vi "Station Config.vi"(8 "error in":errorcluster) -> (0 "error out":errorcluster)   [LabVIEW 2025, in "Full User Interface.lvlib"]
uses:
  Full User Interface.lvlib
  Station Config.ctl
  Station Info.ctl
  Localization/Section.ctl
  Localization/Localization.lvlib
panel:
  in  "Cancel":bool
  in  "OK":bool
  in  "Tree":string(tree)
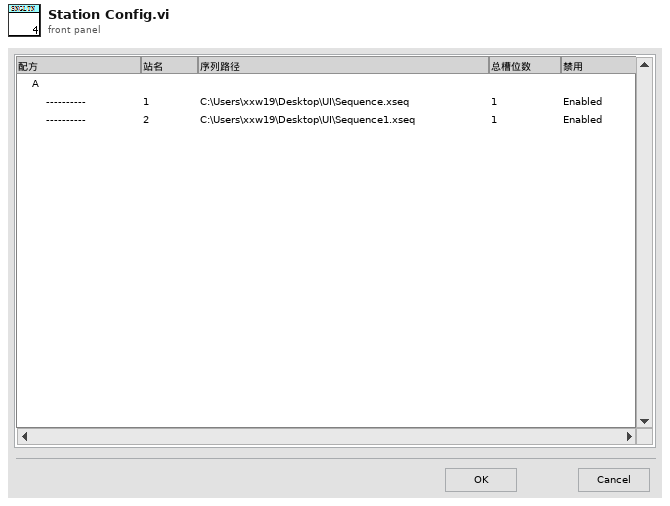
[diagram p1: front panel]
types:
  T1 = enum32{"Invalid", "Standard", "Closed", "Hidden", "Minimized", "Maximized"}
  T2 = enum32{"invalid app kind", "Development System", "Run Time System", "Student Edition", "Embedded LabVIEW", "Evaluation", "Custom"}
  T3 = typedef "Localization.lvlib/Section.ctl" = enum16{"Menu", "Title", "Workstation Config", "TestInterface"}
  T4 = cluster{"Navigate Tree:Get Parent":string, "Tag":string, "Col":i32}
  T5 = typedef "LVPoint32TypeDef.ctl" = cluster{"Horizontal":i32, "Vertical":i32}
  T6 = typedef "Full User Interface.lvlib/Station Config.ctl" = map{string, map{i32, T7}}
  T7 = typedef "Full User Interface.lvlib/Station Info.ctl" = cluster{"SeqFilename":path, "NumberOfSocket":i32, "Disable":bool}
  T8 = cluster{"Core":cluster{"Current VI Reference":refnum<vi>, "Close Panel on Exit?":bool}, "Tree":refnum<vi>, "Station Config":T6, "variant":variant, "clipboard":map{i32, T7}}
  T9 = cluster{"Current VI Reference":refnum<vi>, "Close Panel on Exit?":bool}
  T10 = cluster{"Left Cell String":string, "Child Text":string[], "Child Tag":string, "Item Indent":i32, "Child Only?":bool, "Glyph Index":i32}[]
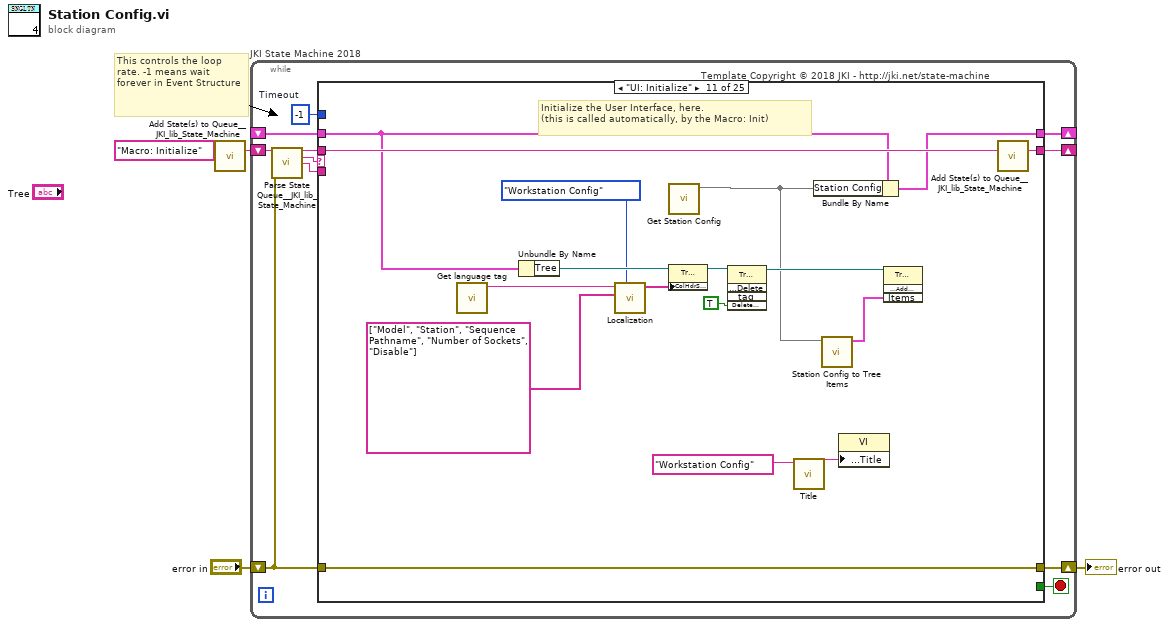
[diagram p0: block diagram]
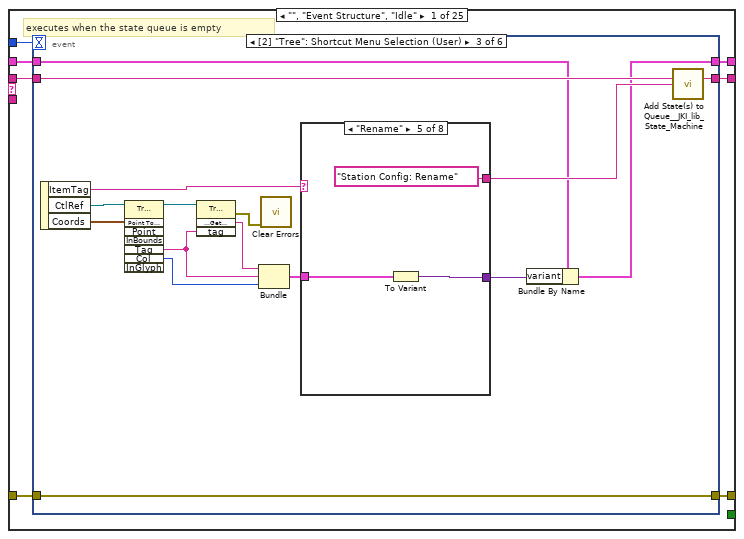
[diagram p2: hidden frame]
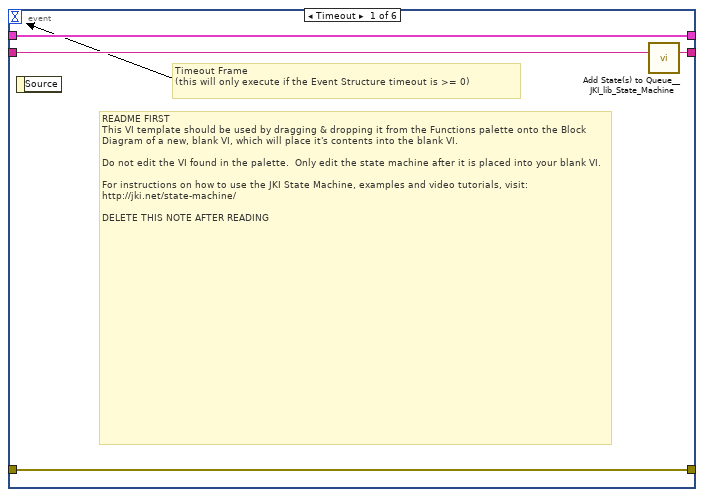
[diagram p3: hidden frame]
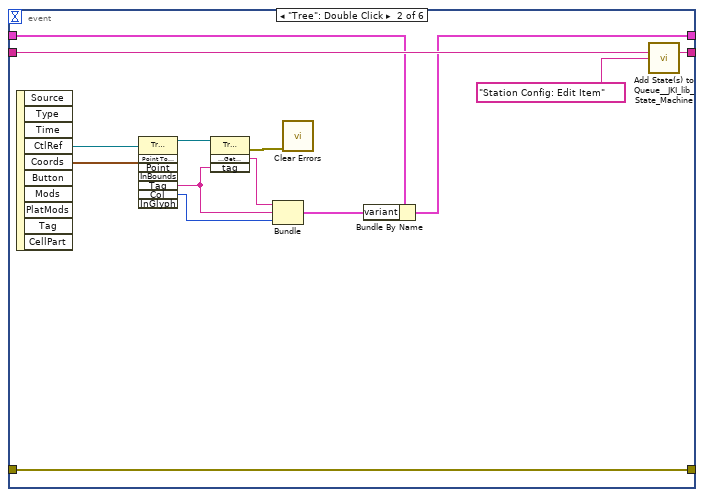
[diagram p4: hidden frame]
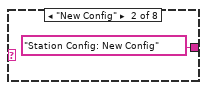
[diagram p6: hidden frame]
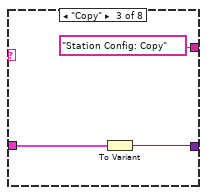
[diagram p7: hidden frame]
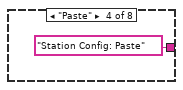
[diagram p8: hidden frame]
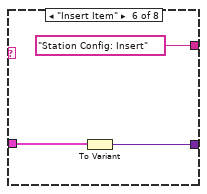
[diagram p9: hidden frame]
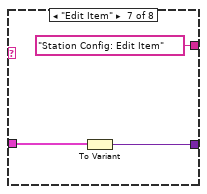
[diagram p10: hidden frame]
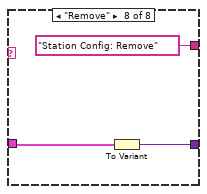
[diagram p11: hidden frame]
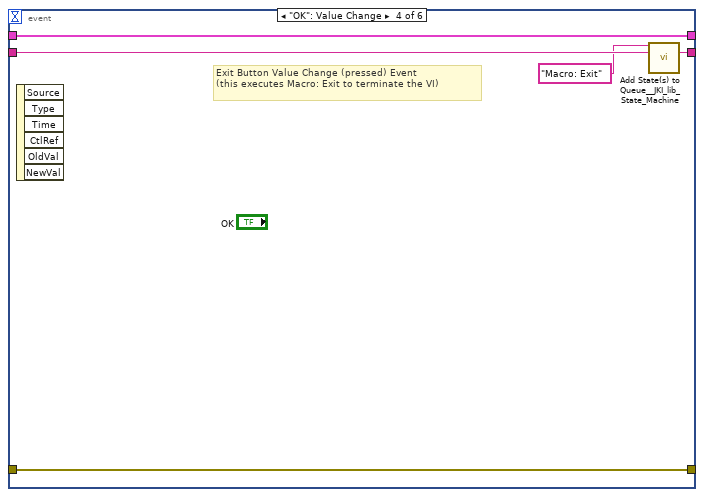
[diagram p12: hidden frame]
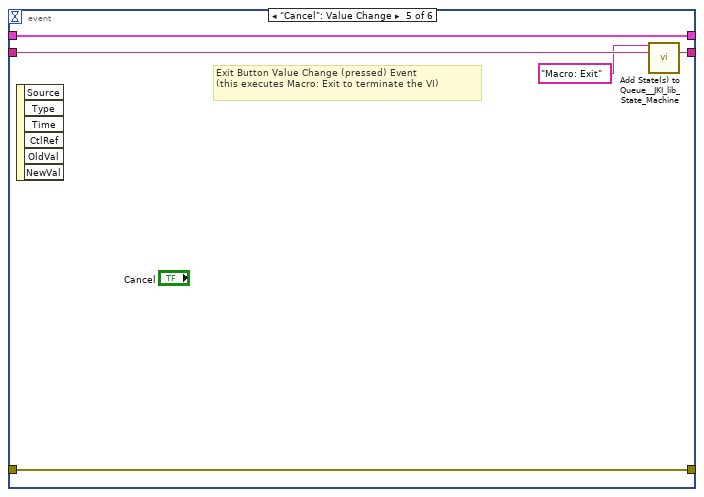
[diagram p13: hidden frame]
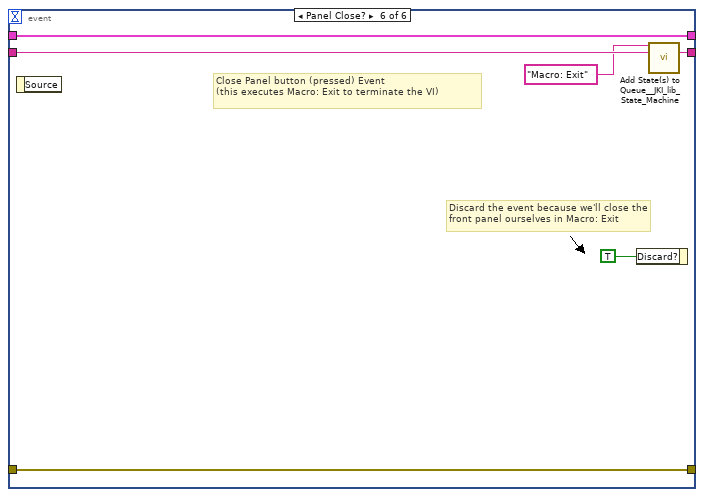
[diagram p14: hidden frame]
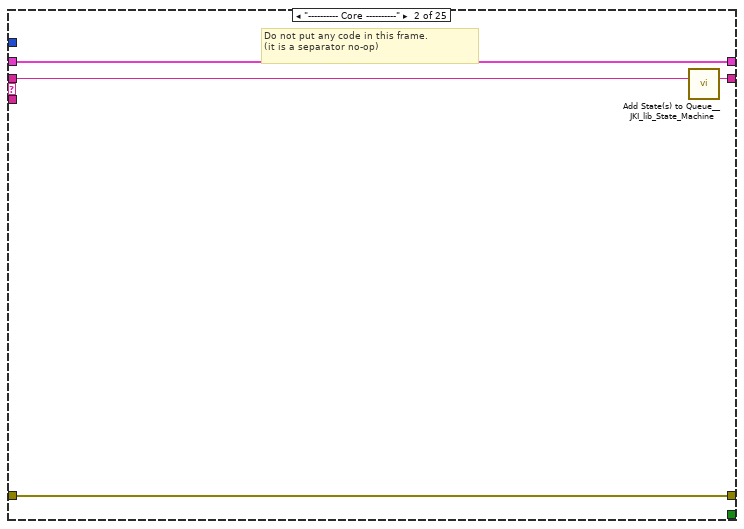
[diagram p15: hidden frame]
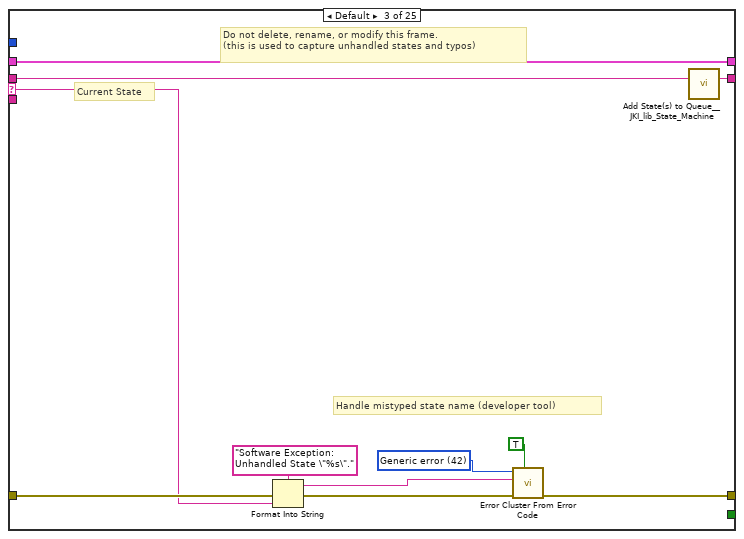
[diagram p16: hidden frame]
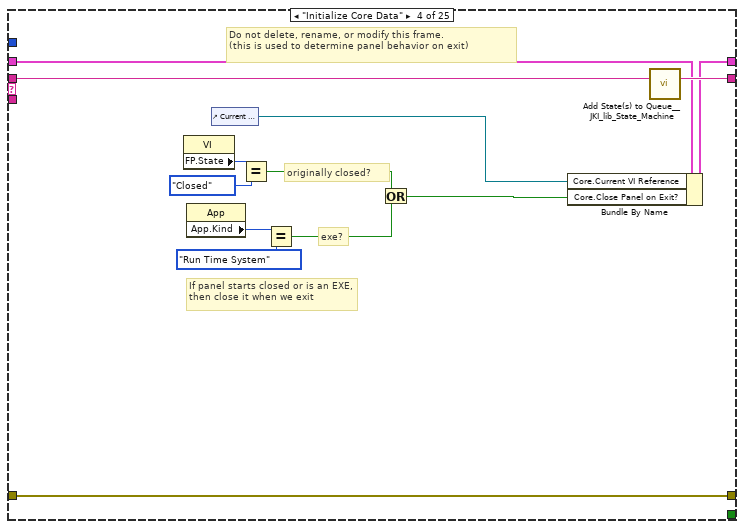
[diagram p17: hidden frame]
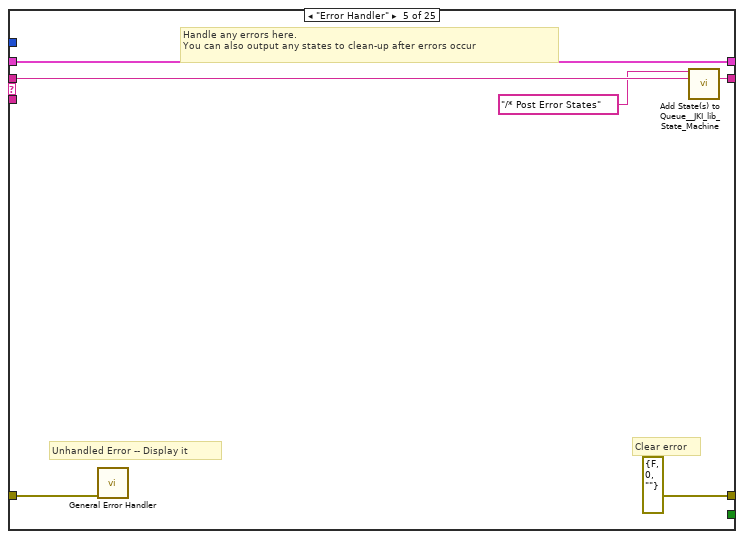
[diagram p18: hidden frame]
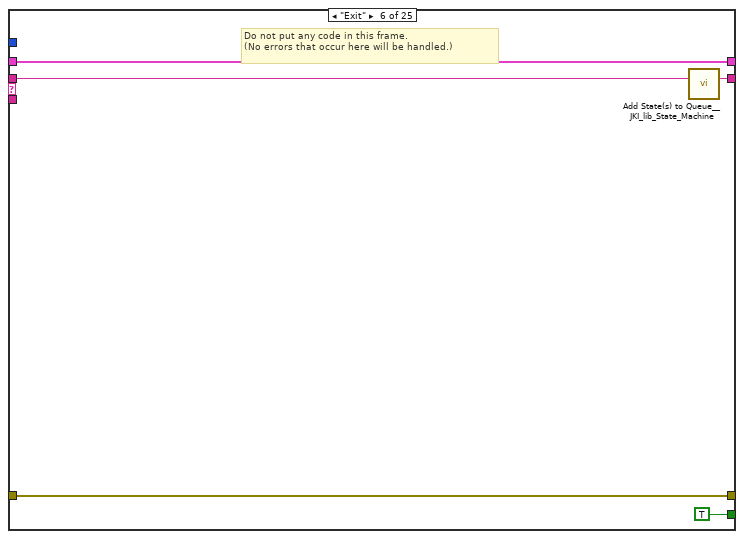
[diagram p19: hidden frame]
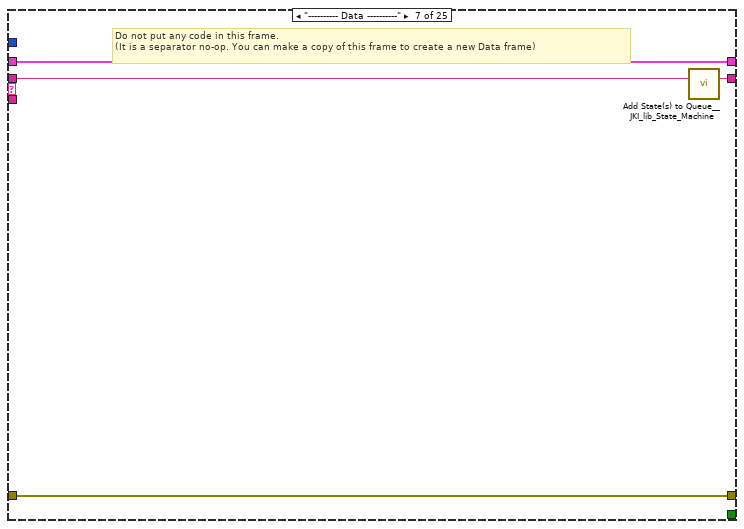
[diagram p20: hidden frame]
diagram:
  # "This controls the loop rate. -1 means wait forever in Event Structure"
  n1 = call <vilib>:"Add State(s) to Queue__JKI_lib_State_Machine.vi"("State(s) in (\"\")"="Macro: Initialize") -> ("States Out"=w4:string)  [unwired: 14 in]
  n2 = while "JKI State Machine 2018" {
    shift-right: [w8] -> _
    shift-left: _ -> [w7]
    shift-right: [w11] -> w1
    shift-left: "error in" -> [w5]
    shift-right: [w10] -> _
    shift-left: w4 -> [w12]
    stop <- w9 stop-if-true
    w6 = -1  # Timeout
    # "Template Copyright © 2018 JKI - http://jki.net/state-machine"
    n3 = call <vilib>:"Parse State Queue__JKI_lib_State_Machine.vi"("State Queue"=w12, "Error In (no error)"=w5) -> ("Remaining States"=w14:string, "Current State"=w15:string, "Arguments"=w13:string)  [unwired: 11 in]
    n4 = case shown="\"UI: Initialize\"" w15 {
      selector: w15 -> [_ _ w94 _ _ _ _ _ _ _ _ _ _ _ _ _ _ _ _ _ _ _ _ _ _]
      tunnel: w14 -> [w22 w93 w98 w117 w123 w128 w132 w141 w147 w151 w168 w174 w185 w254 w259 w269 w273 w280 w288 w303 w319 w335 w345 w354 w377]
      tunnel: w13 -> [_ _ _ _ _ _ _ _ _ _ _ w169 w179 _ _ _ _ _ _ _ _ _ _ _ _]
      tunnel: w7 -> [w20 w90 w96 w110 w120 w126 w129 _ w142 w148 w162 w172 w181 w251 w256 w266 w270 w277 w284 w292 w308 w328 w338 w349 w369]
      tunnel: [w19 w91 w100 w114 errorcluster {"status"=FALSE, "code"=0, "source"=""} ("error out") w125 w130 w138 w143 w149 w166 w170 w182 w252 w257 w267 w271 w275 w286 w301 w317 w333 w343 w352 w375] -> w11
      tunnel: w5 -> [w18 w91 w99 w114 w119 w125 w130 w138 w144 w149 w166 w171 w183 w252 w257 w267 w271 w278 w286 w301 w317 w333 w343 w352 w375]
      tunnel: [w21 w92 w97 w116 w122 w127 w131 w140 w146 w150 w167 w173 w184 w253 w258 w268 w272 w279 w287 w302 w318 w334 w344 w353 w376] -> w10
      tunnel: [_ _ _ _ _ TRUE _ _ _ _ _ _ _ _ _ _ _ _ _ _ _ _ _ _ _] -> w9
      tunnel: [w17 w90 w96 w115 w120 w126 w129 w139 w142 w148 w160 w172 w181 w251 w256 w266 w270 w277 w282 w290 w306 w326 w336 w348 w367] -> w8
      tunnel: w6 -> [w16 _ _ _ _ _ _ _ _ _ _ _ _ _ _ _ _ _ _ _ _ _ _ _ _]
      frame "", "Event Structure", "Idle" {
        # "executes when the state queue is empty"
        n5 = event shown="[2] \"Tree\": Shortcut Menu Selection (User)" {
          selector: _ -> [_ _ _ _ _ _]
          dyn-events: _ -> [_ _ _ _ _ _]
          timeout: w16 -> [_ _ _ _ _ _]
          tunnel: w22 -> [w26 w40 w56 w78 w83 w89]
          tunnel: [w25 w39 w55 w77 w82 w88] -> w21
          tunnel: w20 -> [w23 w29 w47 w75 w80 w86]
          tunnel: [w24 w38 w54 w76 w81 w87] -> w19
          tunnel: w18 -> [w24 w38 w54 w76 w81 w87]
          tunnel: [w23 w28 w46 w75 w80 w86] -> w17
          event Timeout {
            # "README FIRST\nThis VI template should be used by dragging & dropping it from the Functions palette onto the Block Diagram of a new, blank VI, which will place it's contents into the blank VI.\n\nDo not edit the VI found in the palette.  Only edit the state machine after it is placed into your blank VI.\n\nFor instructions on how to use the JKI State Machine, examples and video tutorials, visit:\nhttp://jki.net/state-machine/\n\nDELETE THIS NOTE AFTER READING"
            # "Timeout Frame\n(this will only execute if the Event Structure timeout is >= 0)"
            n6 = event-data() -> ()  [unwired: 1 in, 1 out]
            n7 = call <vilib>:"Add State(s) to Queue__JKI_lib_State_Machine.vi"("State(s) in (\"\")"=w26) -> ("States Out"=w25:string)  [unwired: 14 in]
          }
          event "Tree": Double Click {
            n8 = event-data() -> ("CtlRef"=w32:refnum<vi>, "Coords"=w31:T5)  [unwired: 1 in, 8 out]
            n9 = invoke class="Tree (strict)" method="Point To Row Column"(reference=w32, "Point"=w31) -> (reference out=w36:refnum<vi>, "Tag"=w35:string, "Col"=w37:i32)  [unwired: 6 in, 5 out]
            n10 = invoke class="Tree (strict)" method="Navigate Tree.Get Parent"(reference=w36, "tag"=w35) -> (error out=w33:errorcluster, "Navigate Tree:Get Parent"=w34:string)  [unwired: 2 in, 2 out]
            n11 = Bundle("Navigate Tree:Get Parent"=w34, "Tag"=w35, "Col"=w37) -> (w30:T4)  [unwired: 1 in]
            n12 = call <vilib>:"Clear Errors.vi"("error in (no error)"=w33) -> ()  [unwired: 5 in, 2 out]
            n13 = Bundle By Name(cluster=w29, "variant"=w30) -> (w28:T8)
            n14 = call <vilib>:"Add State(s) to Queue__JKI_lib_State_Machine.vi"("State(s) in (\"\")"=w40, "State(s) at Back (\"\")"="Station Config: Edit Item" ("State(s) at Back (\"\")")) -> ("States Out"=w39:string)  [unwired: 13 in]
          }
          event "Tree": Shortcut Menu Selection (User) {
            n15 = event-data() -> ("ItemTag"=w53:string, "CtlRef"=w52:refnum<vi>, "Coords"=w51:T5)  [unwired: 1 in]
            n16 = invoke class="Tree (strict)" method="Point To Row Column"(reference=w52, "Point"=w51) -> (reference out=w44:refnum<vi>, "Tag"=w43:string, "Col"=w49:i32)  [unwired: 6 in, 5 out]
            n17 = invoke class="Tree (strict)" method="Navigate Tree.Get Parent"(reference=w44, "tag"=w43) -> (error out=w41:errorcluster, "Navigate Tree:Get Parent"=w42:string)  [unwired: 2 in, 2 out]
            n18 = Bundle("Navigate Tree:Get Parent"=w42, "Tag"=w43, "Col"=w49) -> (w48:T4)  [unwired: 1 in]
            n19 = call <vilib>:"Clear Errors.vi"("error in (no error)"=w41) -> ()  [unwired: 5 in, 2 out]
            n20 = case shown="\"Rename\"" w53 {
              tunnel: [_ "Station Config: New Config" "Station Config: Copy" "Station Config: Paste" "Station Config: Rename" "Station Config: Insert" "Station Config: Edit Item" "Station Config: Remove"] -> w50
              tunnel: w48 -> [_ _ w59 _ w63 w66 w69 w72]
              tunnel: [_ _ w58 _ w62 w65 w68 w71] -> w45
              frame Default {
              }
              frame "New Config" {
              }
              frame "Copy" {
                n21 = To Variant(anything=w59) -> (Variant=w58:variant)
              }
              frame "Paste" {
              }
              frame "Rename" {
                n22 = To Variant(anything=w63) -> (Variant=w62:variant)
              }
              frame "Insert Item" {
                n23 = To Variant(anything=w66) -> (Variant=w65:variant)
              }
              frame "Edit Item" {
                n24 = To Variant(anything=w69) -> (Variant=w68:variant)
              }
              frame "Remove" {
                n25 = To Variant(anything=w72) -> (Variant=w71:variant)
              }
            }
            n26 = Bundle By Name(cluster=w47, "variant"=w45) -> (w46:T8)
            n27 = call <vilib>:"Add State(s) to Queue__JKI_lib_State_Machine.vi"("State(s) in (\"\")"=w56, "State(s) at Back (\"\")"=w50) -> ("States Out"=w55:string)  [unwired: 13 in]
          }
          event "OK": Value Change {
            # "Exit Button Value Change (pressed) Event\n(this executes Macro: Exit to terminate the VI)"
            n28 = event-data() -> ()  [unwired: 1 in, 6 out]
            n29 = call <vilib>:"Add State(s) to Queue__JKI_lib_State_Machine.vi"("State(s) in Front (\"\")"="Macro: Exit", "State(s) in (\"\")"=w78) -> ("States Out"=w77:string)  [unwired: 13 in]
          }
          event "Cancel": Value Change {
            # "Exit Button Value Change (pressed) Event\n(this executes Macro: Exit to terminate the VI)"
            n30 = event-data() -> ()  [unwired: 1 in, 6 out]
            n31 = call <vilib>:"Add State(s) to Queue__JKI_lib_State_Machine.vi"("State(s) in Front (\"\")"="Macro: Exit", "State(s) in (\"\")"=w83) -> ("States Out"=w82:string)  [unwired: 13 in]
          }
          event Panel Close? {
            # "Discard the event because we'll close the front panel ourselves in Macro: Exit"
            # "Close Panel button (pressed) Event\n(this executes Macro: Exit to terminate the VI)"
            n32 = event-data() -> ()  [unwired: 1 in, 1 out]
            n33 = event-data("Discard?"=TRUE) -> ()  [unwired: 1 in, 1 out]
            n34 = call <vilib>:"Add State(s) to Queue__JKI_lib_State_Machine.vi"("State(s) in Front (\"\")"="Macro: Exit", "State(s) in (\"\")"=w89) -> ("States Out"=w88:string)  [unwired: 13 in]
          }
        }
      }
      frame "---------- Core ----------" {
        # "Do not put any code in this frame.\n(it is a separator no-op)"
        n35 = call <vilib>:"Add State(s) to Queue__JKI_lib_State_Machine.vi"("State(s) in (\"\")"=w93) -> ("States Out"=w92:string)  [unwired: 14 in]
      }
      frame Default {
        w103 = 42 items=["No error", "Argument error", "Memory is full", "Out of zone", "End of file", "File already open", "Generic file I/O error", "File not found", "File permission error", "Disk is full", "Duplicate path", "Too many files open", "System feature not enabled", "Resource file not found", "Cannot add resource", "Resource not found", "Image not found", "Image memory error", "Pen does not exist", "Config type invalid", "Config token not found", "Config parse error", "Config memory error", "Bad external code format", "Bad external code offset", "External code not present", "Null window", "Destroy window error", "Null menu", "Print aborted", "Bad print record", "Print driver error", "Windows error during printing", "Memory error during printing", "Print dialog error", "Generic print error", "Invalid device refnum", "Device not found", "Device parameter error", "Device unit error", "Cannot open device", "Device call aborted", "Generic error", "Cancelled by user", "Object ID too low", "Object ID too high", "Object not in heap", "Unknown heap", "Unknown object (invalid DefProc)", "Unknown object (DefProc not in table)", "Message out of range", "Invalid (null) method", "Unknown message", "Manager call not supported", "Bad address", "Network operation in progress", "Network operation timed out", "Connection is busy", "Network attribute not supported", "Network error", "Address in use", "System out of memory", "Connection aborted", "Connection refused", "Not connected", "Already connected", "Connection closed", "Initialization error (interapplication manager)", "Bad occurrence", "Wait on unbound occurrence handler", "Occurrence queue overflow", "Datalog type conflict", "Unused", "Unrecognized type (interapplication manager)", "Memory corrupt", "Failed to make temporary DLL", "Old CIN version", "Drag socket not found", "Failed to load drop-object", "Failed to register OLE object", "Failed to release OLE object", "Format specifier type mismatch", "Unknown format specifier", "Too few format specifiers", "Too many format specifiers", "Scan failed", "Newer CIN version", "Error converting to variant", "Runtime menu error", "Password tampered", "Variant attribute not found", "Incompatible variant data type", "Event data is not available", "Event Store is not present", "Occurrence is not found", "Event Queue is not created", "Event info is not available", "Refnum passed is NULL", "Error retrieving Class GUID", "Error retrieving CoClass GUID", "Error retrieving TypeLib GUID.", "Bad built application magic bytes.", "Specific driver is different from the specific driver associated with the Logical Name.", "There is no session opened to the class driver.", "Max Error", "MAX - Error with config objects", "MAX - Error loading configuration", "MAX - Group not supported"]
        # "Current State"
        # "Do not delete, rename, or modify this frame.\n(this is used to capture unhandled states and typos)"
        # "Handle mistyped state name (developer tool)"
        n36 = Format Into String(format string="Software Exception: Unhandled State \"%s\"." ("message"), error in=w99, w94) -> (resulting string=w102:string, error out=w101:errorcluster)  [unwired: 1 in]
        n37 = call <vilib>:"Error Cluster From Error Code.vi"("show call chain? (False)"=TRUE, "error in (no error)"=w101, "error message (\"\")"=w102, "error code (0)"=w103) -> ("error out"=w100:errorcluster)  [unwired: 5 in]
        n38 = call <vilib>:"Add State(s) to Queue__JKI_lib_State_Machine.vi"("State(s) in (\"\")"=w98) -> ("States Out"=w97:string)  [unwired: 14 in]
      }
      frame "Initialize Core Data" {
        # "Do not delete, rename, or modify this frame.\n(this is used to determine panel behavior on exit)"
        # "originally closed?"
        # "exe?"
        # "If panel starts closed or is an EXE, then close it when we exit"
        n39 = property class="VI"() -> ("FP.State"=w107:T1)  [unwired: 2 in, 2 out]
        n40 = property class="App"() -> ("App.Kind"=w113:T2)  [unwired: 2 in, 2 out]
        n41 = control-ref of="Current VI Reference"() -> (w108:refnum<vi>)
        n42 = Equal?(x=w107, y=T1."Closed" ("Front Panel Window:State")) -> (x = y?=w105:bool)
        n43 = Equal?(x=w113, y=T2."Run Time System" ("Application:Kind")) -> (x = y?=w111:bool)
        n44 = Or(x=w105, y=w111) -> (x .or. y?=w109:bool)
        n45 = Bundle By Name(cluster=w110, "Core.Current VI Reference"=w108, "Core.Close Panel on Exit?"=w109) -> (w115:T8)
        n46 = call <vilib>:"Add State(s) to Queue__JKI_lib_State_Machine.vi"("State(s) in (\"\")"=w117) -> ("States Out"=w116:string)  [unwired: 14 in]
      }
      frame "Error Handler" {
        # "Unhandled Error -- Display it"
        # "Handle any errors here.\nYou can also output any states to clean-up after errors occur"
        # "Clear error"
        n47 = call <vilib>:"General Error Handler.vi"("error in (no error)"=w119) -> ()  [unwired: 10 in, 5 out]
        n48 = call <vilib>:"Add State(s) to Queue__JKI_lib_State_Machine.vi"("State(s) in Front (\"\")"="/* Post Error States", "State(s) in (\"\")"=w123) -> ("States Out"=w122:string)  [unwired: 13 in]
      }
      frame "Exit" {
        # "Do not put any code in this frame.\n(No errors that occur here will be handled.)"
        n49 = call <vilib>:"Add State(s) to Queue__JKI_lib_State_Machine.vi"("State(s) in (\"\")"=w128) -> ("States Out"=w127:string)  [unwired: 14 in]
      }
      frame "---------- Data ----------" {
        # "Do not put any code in this frame.\n(It is a separator no-op. You can make a copy of this frame to create a new Data frame)"
        n50 = call <vilib>:"Add State(s) to Queue__JKI_lib_State_Machine.vi"("State(s) in (\"\")"=w132) -> ("States Out"=w131:string)  [unwired: 14 in]
      }
      frame "Data: Initialize" {
        w133 = map{i32, T7} {}  # clipboard
        w134 = variant  # variant
        w135 = T6 {}  # Station Config
        w137 = T9 {"Current VI Reference"=refnum, "Close Panel on Exit?"=FALSE}  # Core
        # "Data names and types of shift register data are defined by this bundle."
        # "Initialize the shift-register data, here.\n(data names are defined by what you wire into the bundle function)"
        n51 = control-ref of="Tree"() -> (w136:refnum<vi>)
        n52 = Bundle("Core"=w137, "Tree"=w136, "Station Config"=w135, "variant"=w134, "clipboard"=w133) -> (w139:T8)  [unwired: 1 in]
        n53 = call <vilib>:"Add State(s) to Queue__JKI_lib_State_Machine.vi"("State(s) in (\"\")"=w141) -> ("States Out"=w140:string)  [unwired: 14 in]
      }
      frame "Data: Cleanup" {
        # "Cleanup any data and references, here.\n(this is called automatically, by the Macro: Exit)"
        n54 = Unbundle By Name(w142) -> ("Core.Current VI Reference"=w145:refnum<vi>)
        n55 = Close Reference(reference=w145, error in (no error)=w144) -> (error out=w143:errorcluster)
        n56 = call <vilib>:"Add State(s) to Queue__JKI_lib_State_Machine.vi"("State(s) in (\"\")"=w147) -> ("States Out"=w146:string)  [unwired: 14 in]
      }
      frame "---------- UI ----------" {
        # "Do not put any code in this frame.\n(It is a separator no-op. You can make a copy of this frame to create a new UI frame)"
        n57 = call <vilib>:"Add State(s) to Queue__JKI_lib_State_Machine.vi"("State(s) in (\"\")"=w151) -> ("States Out"=w150:string)  [unwired: 14 in]
      }
      frame "UI: Initialize" {
        # "Initialize the User Interface, here.\n(this is called automatically, by the Macro: Init)"
        n58 = call "Get language tag.vi"() -> ("language tag"=w158:string)  [unwired: 11 in]
        n59 = Unbundle By Name(w162) -> ("Tree"=w159:refnum<vi>)
        n60 = call "Localization.vi"("section"=Section."Workstation Config", "key"=string[] ["Model", "Station", "Sequence Pathname", "Number of Sockets", "Disable"], "Language key"=w158) -> ("Value"=w155:string[])  [unwired: 7 in, 1 out]
        n61 = call "Get Station Config.vi"() -> ("Station Config"=w161:T6)  [unwired: 10 in, 1 out]
        n62 = property class="Tree (strict)"(reference=w159, "ColHdrString"=w155) -> (reference out=w154:refnum<vi>)  [unwired: 1 in, 1 out]
        n63 = invoke class="Tree (strict)" method="Edit Tree Items.Delete"(reference=w154, "Delete Children"=TRUE ("Delete Children?")) -> (reference out=w164:refnum<vi>)  [unwired: 3 in, 4 out]
        n64 = call "Title.vi"("Front Panel Window:Title"="Workstation Config") -> ("Title"=w152:string)  [unwired: 10 in]
        n65 = Bundle By Name(cluster=w162, "Station Config"=w161) -> (w160:T8)
        n66 = call "Station Config to Tree Items.vi"("Station Config"=w161) -> ("Tree Items"=w163:T10)  [unwired: 10 in]
        n67 = property on="Property Node" class="VI"("Front Panel.Title"=w152) -> ()  [unwired: 2 in, 2 out]
        n68 = invoke class="Tree (strict)" method="Edit Tree Items.Add Multiple Items to End"(reference=w164, "Items"=w163) -> ()  [unwired: 2 in, 4 out]
        n69 = call <vilib>:"Add State(s) to Queue__JKI_lib_State_Machine.vi"("State(s) in (\"\")"=w168) -> ("States Out"=w167:string)  [unwired: 14 in]
      }
      frame "UI: Cursor Set" {
        # "Argument"
        # "Set and Unset Cursor Busy.\n(Usage: \"UI: Cursor Set >> Busy|Idle\")"
        n70 = case shown="\"Idle\", Default" w169 {
          tunnel: w171 -> [w176 w178]
          tunnel: [w175 w177] -> w170
          frame "Idle", Default {
            n71 = call <vilib>:"Unset Busy.vi"("error in (no error)"=w176) -> ("error out"=w175:errorcluster)  [unwired: 10 in]
          }
          frame "Busy" {
            n72 = call <vilib>:"Set Busy.vi"("error in (no error)"=w178) -> ("error out"=w177:errorcluster)  [unwired: 9 in, 1 out]
          }
        }
        n73 = call <vilib>:"Add State(s) to Queue__JKI_lib_State_Machine.vi"("State(s) in (\"\")"=w174) -> ("States Out"=w173:string)  [unwired: 14 in]
      }
      frame "UI: Front Panel State" {
        # "Argument"
        # "Set Front Panel Open or Closed\n(Usage: \"UI: Front Panel State >> Open|Close\")"
        n74 = Unbundle By Name(w181) -> ("Core.Current VI Reference"=w180:refnum<vi>)
        n75 = case shown="\"Minimize\", \"Minimized\"" w179 {
          tunnel: w183 -> [w191 w206 w217 w230 w243]
          tunnel: [w193 w207 w219 w232 w245] -> w182
          tunnel: w180 -> [w192 w204 w218 w231 w244]
          frame "Open", "Standard", Default {
            w186 = T1."Standard" ("State")
            n76 = property class="VI"(reference=w192, error in=w191) -> (reference out=w189:refnum<vi>, error out=w190:errorcluster, "FP.State"=w188:T1)
            n77 = Not Equal?(x=w188, y=w186) -> (x != y?=w187:bool)
            n78 = case shown="True" w187 {
              tunnel: [w197 w199] -> w193
              tunnel: w190 -> [w196 w199]
              tunnel: w189 -> [w195 _]
              tunnel: w186 -> [w194 _]
              frame True {
                n79 = invoke class="VI" method="FP.Open"(reference=w195, error in=w196, "Activate"=TRUE, "State"=w194) -> (error out=w197:errorcluster)  [unwired: 1 in, 4 out]
              }
              frame False {
              }
            }
          }
          frame "Close", "Closed" {
            n80 = property class="VI"(reference=w204, error in=w206) -> (reference out=w203:refnum<vi>, error out=w205:errorcluster, "FP.State"=w201:T1)
            n81 = Not Equal?(x=w201, y=T1."Closed" ("Front Panel Window:State")) -> (x != y?=w200:bool)
            n82 = case shown="True" w200 {
              tunnel: [w208 w211] -> w207
              tunnel: w205 -> [w208 w210]
              tunnel: w203 -> [_ w209]
              frame False {
              }
              frame True {
                n83 = invoke class="VI" method="FP.Close"(reference=w209, error in=w210) -> (error out=w211:errorcluster)  [unwired: 1 in, 2 out]
              }
            }
          }
          frame "Hidden", "Hide" {
            w212 = T1."Hidden" ("State")
            n84 = property class="VI"(reference=w218, error in=w217) -> (reference out=w215:refnum<vi>, error out=w216:errorcluster, "FP.State"=w214:T1)
            n85 = Not Equal?(x=w214, y=w212) -> (x != y?=w213:bool)
            n86 = case shown="True" w213 {
              tunnel: [w223 w224] -> w219
              tunnel: w216 -> [w222 w224]
              tunnel: w215 -> [w221 _]
              tunnel: w212 -> [w220 _]
              frame True {
                n87 = invoke class="VI" method="FP.Open"(reference=w221, error in=w222, "State"=w220) -> (error out=w223:errorcluster)  [unwired: 2 in, 4 out]
              }
              frame False {
              }
            }
          }
          frame "Minimize", "Minimized" {
            w225 = T1."Minimized" ("State")
            n88 = property class="VI"(reference=w231, error in=w230) -> (reference out=w228:refnum<vi>, error out=w229:errorcluster, "FP.State"=w227:T1)
            n89 = Not Equal?(x=w227, y=w225) -> (x != y?=w226:bool)
            n90 = case shown="True" w226 {
              tunnel: [w236 w237] -> w232
              tunnel: w229 -> [w235 w237]
              tunnel: w228 -> [w234 _]
              tunnel: w225 -> [w233 _]
              frame True {
                n91 = invoke class="VI" method="FP.Open"(reference=w234, error in=w235, "State"=w233) -> (error out=w236:errorcluster)  [unwired: 2 in, 4 out]
              }
              frame False {
              }
            }
          }
          frame "Maximize", "Maximized" {
            w238 = T1."Maximized" ("State")
            n92 = property class="VI"(reference=w244, error in=w243) -> (reference out=w241:refnum<vi>, error out=w242:errorcluster, "FP.State"=w240:T1)
            n93 = Not Equal?(x=w240, y=w238) -> (x != y?=w239:bool)
            n94 = case shown="True" w239 {
              tunnel: [w249 w250] -> w245
              tunnel: w242 -> [w248 w250]
              tunnel: w241 -> [w247 _]
              tunnel: w238 -> [w246 _]
              frame True {
                n95 = invoke class="VI" method="FP.Open"(reference=w247, error in=w248, "State"=w246) -> (error out=w249:errorcluster)  [unwired: 2 in, 4 out]
              }
              frame False {
              }
            }
          }
        }
        n96 = call <vilib>:"Add State(s) to Queue__JKI_lib_State_Machine.vi"("State(s) in (\"\")"=w185) -> ("States Out"=w184:string)  [unwired: 14 in]
      }
      frame "---------- Macro ----------" {
        # "Do not put any code in this frame.\n(It is a separator no-op. You can make a copy of this frame to create a new Macro frame)"
        n97 = call <vilib>:"Add State(s) to Queue__JKI_lib_State_Machine.vi"("State(s) in (\"\")"=w254) -> ("States Out"=w253:string)  [unwired: 14 in]
      }
      frame "Macro: Initialize" {
        w255 = "Data: Initialize\nInitialize Core Data\nUI: Initialize\nUI: Front Panel State >> Open"  # Data: Initialize Initialize Core Data UI: Initialize UI: Front Panel State >> Open
        # "Initialization Macro\n(This is called once, when the VI starts)"
        n98 = call <vilib>:"Add State(s) to Queue__JKI_lib_State_Machine.vi"("State(s) in Front (\"\")"=w255, "State(s) in (\"\")"=w259) -> ("States Out"=w258:string)  [unwired: 13 in]
      }
      frame "Macro: Exit" {
        # "Exit Macro\n(This is called once, when the VI exits)"
        n99 = Unbundle By Name(w266) -> ("Core.Close Panel on Exit?"=w265:bool)
        n100 = Select(t="UI: Front Panel State >> Close", s=w265, f="") -> (s? t:f=w262:string)
        n101 = call <vilib>:"Add State(s) to Queue__JKI_lib_State_Machine.vi"("State(s) in (\"\")"=w262, "State(s) at Back (\"\")"="Data: Cleanup\nExit") -> ("States Out"=w260:string)  [unwired: 13 in]
        n102 = call <vilib>:"Add State(s) to Queue__JKI_lib_State_Machine.vi"("State(s) in Front (\"\")"=w260, "State(s) in (\"\")"=w269) -> ("States Out"=w268:string)  [unwired: 13 in]
      }
      frame "---------- Station Config ----------" {
        # "Template Separator\n(You can make a copy of, or modify, this frame)"
        n103 = call <vilib>:"Add State(s) to Queue__JKI_lib_State_Machine.vi"("State(s) in (\"\")"=w273) -> ("States Out"=w272:string)  [unwired: 14 in]
      }
      frame "Station Config: Save" {
        # "Template Separator\n(You can make a copy of, or modify, this frame)"
        n104 = Unbundle By Name(w277) -> ("Station Config"=w276:T6)
        n105 = call "Set Station Config.vi"("Station Config"=w276) -> ("error out"=w274:errorcluster)  [unwired: 10 in]
        n106 = Merge Errors(w274, w278) -> (w275:errorcluster)
        n107 = call <vilib>:"Add State(s) to Queue__JKI_lib_State_Machine.vi"("State(s) in (\"\")"=w280) -> ("States Out"=w279:string)  [unwired: 14 in]
      }
      frame "Station Config: New Config" {
        # "Template Separator\n(You can make a copy of, or modify, this frame)"
        n108 = Unbundle By Name(w284) -> ("Station Config"=w285:T6)
        n109 = call "New Station Config (Name).vi"("Station Config in"=w285) -> ("Station Config out"=w283:T6)  [unwired: 9 in, 1 out]
        n110 = Bundle By Name(cluster=w284, "Station Config"=w283) -> (w282:T8)
        n111 = call <vilib>:"Add State(s) to Queue__JKI_lib_State_Machine.vi"("State(s) in (\"\")"=w288, "State(s) at Back (\"\")"="Station Config: Save\nUI: Initialize" ("State(s) at Back (\"\")")) -> ("States Out"=w287:string)  [unwired: 13 in]
      }
      frame "Station Config: Insert" {
        # "Your code here.\n(You can make a copy of, or modify, this frame)"
        n112 = Unbundle By Name(w292) -> ("Station Config"=w294:T6, "variant"=w300:variant)
        n113 = Variant To Data(type=T4 {"Navigate Tree:Get Parent"="", "Tag"="", "Col"=0}, Variant=w300) -> (data=w298:T4)  [unwired: 1 in, 1 out]
        n114 = Unbundle(w298) -> ("Navigate Tree:Get Parent"=w295:string, "Tag"=w296:string)  [unwired: 1 out]
        n115 = Empty String/Path?(string/path=w295) -> (empty?=w297:bool)
        n116 = Select(t=w296, s=w297, f=w295) -> (s? t:f=w293:string)
        n117 = call "New Station Config Item.vi"("Key"=w293, "Station Config in"=w294) -> ("Station Config out"=w291:T6)  [unwired: 9 in]
        n118 = Bundle By Name(cluster=w292, "Station Config"=w291) -> (w290:T8)
        n119 = call <vilib>:"Add State(s) to Queue__JKI_lib_State_Machine.vi"("State(s) in (\"\")"=w303, "State(s) at Back (\"\")"="Station Config: Save\nUI: Initialize" ("State(s) at Back (\"\")")) -> ("States Out"=w302:string)  [unwired: 13 in]
      }
      frame "Station Config: Edit Item" {
        # "Template Separator\n(You can make a copy of, or modify, this frame)"
        n120 = Unbundle By Name(w308) -> ("Station Config"=w313:T6, "variant"=w315:variant)
        n121 = Variant To Data(type=T4 {"Navigate Tree:Get Parent"="", "Tag"="", "Col"=0}, Variant=w315) -> (data=w314:T4)  [unwired: 1 in, 1 out]
        n122 = Unbundle(w314) -> ("Navigate Tree:Get Parent"=w305:string, "Tag"=w309:string)  [unwired: 1 out]
        n123 = Empty String/Path?(string/path=w305) -> (empty?=w312:bool)
        n124 = Empty String/Path?(string/path=w309) -> (empty?=w311:bool)
        n125 = Or(x=w312, y=w311) -> (x .or. y?=w310:bool)
        n126 = case shown="False" w310 {
          tunnel: w313 -> [w323 w324]
          tunnel: w309 -> [w321 _]
          tunnel: [w322 w324] -> w307
          tunnel: w305 -> [w320 _]
          frame False {
            n127 = call "Edit Station Config Item.vi"("Key 2"=w321, "Key"=w320, "Station Config in"=w323) -> ("Station Config out"=w322:T6)  [unwired: 8 in]
          }
          frame True {
          }
        }
        n128 = Bundle By Name(cluster=w308, "Station Config"=w307) -> (w306:T8)
        n129 = call <vilib>:"Add State(s) to Queue__JKI_lib_State_Machine.vi"("State(s) in (\"\")"=w319, "State(s) at Back (\"\")"="Station Config: Save\nUI: Initialize" ("State(s) at Back (\"\")")) -> ("States Out"=w318:string)  [unwired: 13 in]
      }
      frame "Station Config: Remove" {
        # "Your code here.\n(You can make a copy of, or modify, this frame)"
        n130 = Unbundle By Name(w328) -> ("Station Config"=w330:T6, "variant"=w331:variant)
        n131 = Variant To Data(type=T4 {"Navigate Tree:Get Parent"="", "Tag"="", "Col"=0}, Variant=w331) -> (data=w329:T4)  [unwired: 1 in, 1 out]
        n132 = call "Remove Station Config Item.vi"("Tag"=w329, "Station Config in"=w330) -> ("Station Config out"=w327:T6)  [unwired: 8 in, 1 out]
        n133 = Bundle By Name(cluster=w328, "Station Config"=w327) -> (w326:T8)
        n134 = call <vilib>:"Add State(s) to Queue__JKI_lib_State_Machine.vi"("State(s) in (\"\")"=w335, "State(s) at Back (\"\")"="Station Config: Save\nUI: Initialize" ("State(s) at Back (\"\")")) -> ("States Out"=w334:string)  [unwired: 13 in]
      }
      frame "Station Config: Copy" {
        # "Template Separator\n(You can make a copy of, or modify, this frame)"
        n135 = Unbundle By Name(w338) -> ("Station Config"=w339:T6, "variant"=w341:variant)
        n136 = Variant To Data(type=T4 {"Navigate Tree:Get Parent"="", "Tag"="", "Col"=0}, Variant=w341) -> (data=w340:T4)  [unwired: 1 in, 1 out]
        n137 = call "Remove Station Config Item.vi"("Tag"=w340, "Station Config in"=w339) -> ("map"=w337:map{i32, T7})  [unwired: 8 in, 1 out]
        n138 = Bundle By Name(cluster=w338, "clipboard"=w337) -> (w336:T8)
        n139 = call <vilib>:"Add State(s) to Queue__JKI_lib_State_Machine.vi"("State(s) in (\"\")"=w345) -> ("States Out"=w344:string)  [unwired: 14 in]
      }
      frame "Station Config: Paste" {
        # "Template Separator\n(You can make a copy of, or modify, this frame)"
        n140 = Unbundle By Name(w349) -> ("Station Config"=w351:T6, "clipboard"=w350:map{i32, T7})
        n141 = Empty Collection?(1:w350) -> (0:w347:bool)
        n142 = case shown="False" w347 {
          tunnel: w351 -> [w360 _]
          tunnel: w350 -> [w359 _]
          tunnel: w349 -> [w358 w361]
          tunnel: [w356 w361] -> w348
          tunnel: ["Station Config: Save\nUI: Initialize" ("State(s) at Back (\"\")") _] -> w346
          frame False {
            n143 = call "New Station Config (Name).vi"("value"=w359, "Station Config in"=w360) -> ("Station Config out"=w357:T6)  [unwired: 8 in, 1 out]
            n144 = Bundle By Name(cluster=w358, "Station Config"=w357) -> (w356:T8)
          }
          frame True {
          }
        }
        n145 = call <vilib>:"Add State(s) to Queue__JKI_lib_State_Machine.vi"("State(s) in (\"\")"=w354, "State(s) at Back (\"\")"=w346) -> ("States Out"=w353:string)  [unwired: 13 in]
      }
      frame "Station Config: Rename" {
        # "Template Separator\n(You can make a copy of, or modify, this frame)"
        n146 = Unbundle By Name(w369) -> ("Station Config"=w371:T6, "variant"=w373:variant)
        n147 = Variant To Data(type=T4 {"Navigate Tree:Get Parent"="", "Tag"="", "Col"=0}, Variant=w373) -> (data=w372:T4)  [unwired: 1 in, 1 out]
        n148 = call "Remove Station Config Item.vi"("Tag"=w372, "Station Config in"=w371) -> ("map"=w366:map{i32, T7}, "Station Config out"=w370:T6)  [unwired: 8 in]
        n149 = Empty Collection?(1:w366) -> (0:w365:bool)
        n150 = call "New Station Config (Name).vi"("value"=w366, "Station Config in"=w370) -> ("Boolean"=w362:bool, "Station Config out"=w368:T6)  [unwired: 8 in]
        n151 = Or(x=w365, y=w362) -> (x .or. y?=w363:bool)
        n152 = case shown="True" w363 {
          tunnel: w369 -> [w381 w382]
          tunnel: w368 -> [w380 _]
          tunnel: [w379 w382] -> w367
          tunnel: ["Station Config: Save\nUI: Initialize" ("State(s) at Back (\"\")") _] -> w364
          frame False {
            n153 = Bundle By Name(cluster=w381, "Station Config"=w380) -> (w379:T8)
          }
          frame True {
          }
        }
        n154 = call <vilib>:"Add State(s) to Queue__JKI_lib_State_Machine.vi"("State(s) in (\"\")"=w377, "State(s) at Back (\"\")"=w364) -> ("States Out"=w376:string)  [unwired: 13 in]
      }
    }
  }
  "error out" <- w1
